vi "Startup.vi"(6 "Config":refnum<class "Config.lvclass">, 7 "Application":refnum<class "Application.lvclass">, 8 "error in (no error)":errorcluster, 9 "Log_Engine":refnum<class "Log_Engine.lvclass">, 10 "DAQ_Engine":refnum<class "DAQ_Engine.lvclass">, 11 "Main in":refnum<class "Main.lvclass">) -> (0 "error out":errorcluster, 3 "Main out":refnum<class "Main.lvclass">, 5 "Application out":refnum<class "Application.lvclass">)   [LabVIEW 2019, in "Main.lvclass"]
doc: "Developed by Kevin Thompson\nkevin@thompsonengineering.net\n\nCopyright 2018\nThompson Engineering, LLC"
uses:
  Main.lvclass
  Config/Config.lvclass
  Application/Application.lvclass
  DAQ_Engine/DAQ_Engine.lvclass
  Log_Engine/Log_Engine.lvclass
  DataTypes/Dependency--cluster.ctl
  Application/Application.lvclass/Application.ctl
  Config/Config.lvclass/Config.ctl
  Main.lvclass/Main.ctl
  Application/Accessors/Get InvWfmsQRef.vi
  Application/Accessors/Get PublicEvents.vi
  Application/Accessors/Get RawDaqDataQRef.vi
  Config/Accessors/Get Main Settings.vi
  Accessors/Set Dependency.vi
  Accessors/Set Settings.vi
  Accessors/Set InvWfmsQRef.vi
  Accessors/Set TerminateAppEvent.vi
  Accessors/Set RawDaqDataQRef.vi
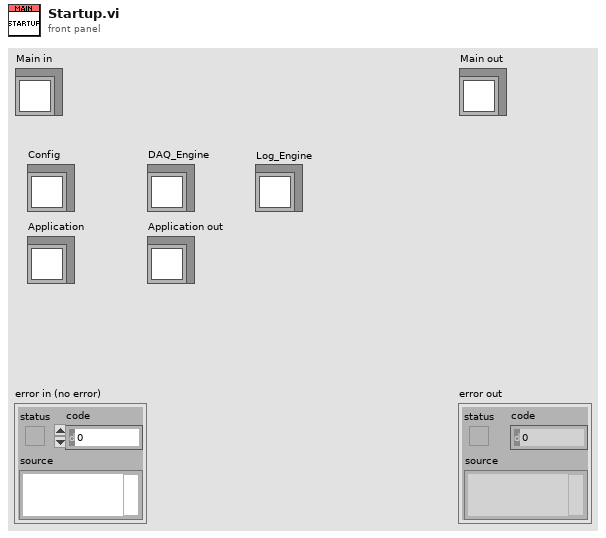
[diagram p1: front panel]
types:
  T1 = typedef "Main.lvclass/Dependency--cluster.ctl" = cluster{"Config":refnum<class "Config.lvclass">, "DAQ":refnum<class "DAQ_Engine.lvclass">, "Log_Engine":refnum<class "Log_Engine.lvclass">}
  T2 = typedef "InverterWaveforms--QRef.ctl" = refnum<queue>
  T3 = typedef "Application.lvclass/Public Events--cluster.ctl" = cluster{"Application.AsyncCmd Event":refnum<user-event>, "Application.AsyncMsg Event":refnum<user-event>, "stop process":refnum<user-event>}
  T4 = typedef "RawDAQDataQRef--cluster.ctl" = refnum<queue>
  T5 = typedef "Main.lvclass/Settings--cluster.ctl" = cluster{"Simulation":bool, "Signal scaling":T6[], "ESR scaling":T7[], "num readings to average":i32[], "ESR alarm threshhold (%)":i32[], "UseDummyVrms":bool, "Dummy Vrms":dbl, "Inverter Database File":path, "default Inverter (name)":string[]}
  T6 = typedef "Main.lvclass/Gain control.ctl" = cluster{"Iin ripple gain":dbl, "Iout ripple gain":dbl, "Iout 60Hz gain ":dbl, "Vout 60Hz gain ":dbl, "Iin ripple offest":dbl, "Iout ripple offset":dbl, "Iout 60Hz offset":dbl, "Vout 60Hz offset":dbl}
  T7 = typedef "Main.lvclass/ESR scaling--cluster.ctl" = cluster{"Gain":dbl, "Offset":dbl}
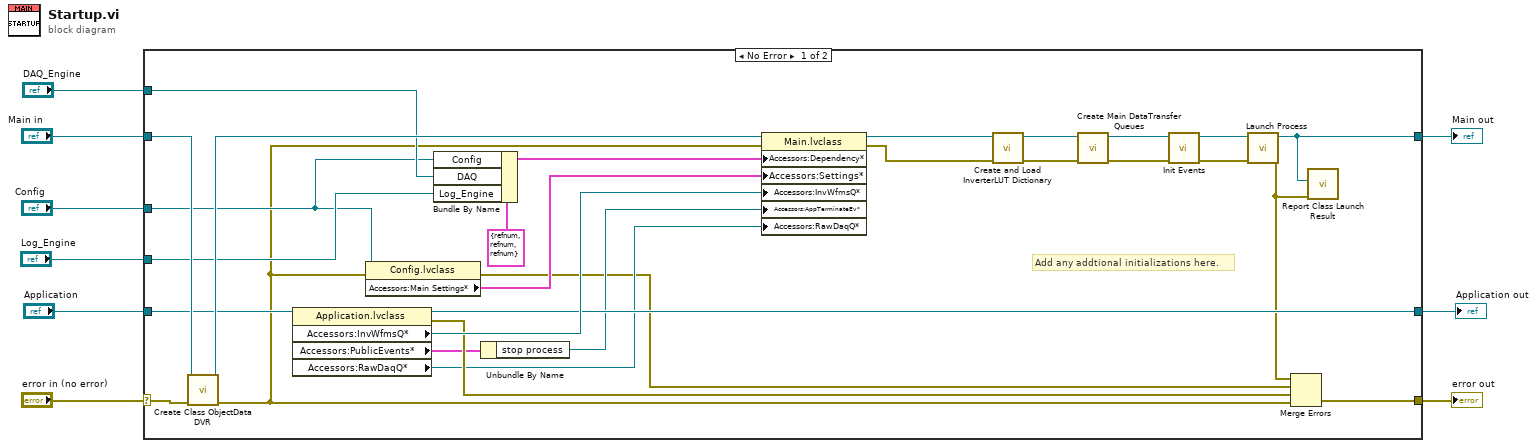
[diagram p0: block diagram]
diagram:
  n1 = case shown="No Error" "error in (no error)" {
    selector: "error in (no error)" -> [w38 w41]
    tunnel: [w35 w41] -> w8
    tunnel: [w24 w40] -> w6
    tunnel: "Main in" -> [w37 w40]
    tunnel: "Config" -> [w19 _]
    tunnel: "Application" -> [w33 w39]
    tunnel: [w30 w39] -> w3
    tunnel: "DAQ_Engine" -> [w28 _]
    tunnel: "Log_Engine" -> [w27 _]
    frame No Error {
      # "Add any addtional initializations here."
      n2 = call "Create Class ObjectData DVR.vi"("error in (no error)"=w38, "Main in"=w37) -> ("error out"=w17:errorcluster, "Main out"=w36:refnum<class "Main.lvclass">)  [unwired: 8 in]
      n3 = property class="Application.lvclass"(reference=w33) -> (reference out=w30:refnum<class "Application.lvclass">, error out=w31:errorcluster, "Accessors:InvWfmsQ*"=w32:T2, "Accessors:PublicEvents*"=w26:T3, "Accessors:RawDaqQ*"=w22:T4)  [unwired: 1 in]
      n4 = property class="Config.lvclass"(reference=w19, error in=w17) -> (error out=w16:errorcluster, "Accessors:Main Settings*"=w18:T5)  [unwired: 1 out]
      n5 = Bundle By Name(cluster=T1 {"Config"=refnum, "DAQ"=refnum, "Log_Engine"=refnum} ("Dependency"), "Config"=w19, "DAQ"=w28, "Log_Engine"=w27) -> (w29:T1)
      n6 = Unbundle By Name(w26) -> ("stop process"=w25:refnum<user-event>)
      n7 = property class="Main.lvclass"(reference=w36, error in=w17, "Accessors:Dependency*"=w29, "Accessors:Settings*"=w18, "Accessors:InvWfmsQ*"=w32, "Accessors:AppTerminateEv*"=w25, "Accessors:RawDaqQ*"=w22) -> (reference out=w13:refnum<class "Main.lvclass">, error out=w11:errorcluster)
      n8 = call "Create and Load InverterLUT Dictionary.vi"("error in (no error)"=w11, "Main.lvclass"=w13) -> ("error out"=w10:errorcluster, "Main out"=w12:refnum<class "Main.lvclass">)  [unwired: 8 in]
      n9 = call "Create Main DataTransfer Queues.vi"("error in (no error)"=w10, "Main in"=w12) -> ("error out"=w20:errorcluster, "Main out"=w21:refnum<class "Main.lvclass">)  [unwired: 6 in, 2 out]
      n10 = call "Init Events.vi"("error in (no error)"=w20, "Main in"=w21) -> ("error out"=w15:errorcluster, "Main out"=w14:refnum<class "Main.lvclass">)  [unwired: 8 in]
      n11 = call "Launch Process.vi"("error in (no error)"=w15, "Main in"=w14) -> ("error out"=w23:errorcluster, "Main out"=w24:refnum<class "Main.lvclass">)  [unwired: 6 in, 2 out]
      n12 = Merge Errors(w23, w16, w31, w17) -> (w35:errorcluster)
      n13 = call "Report Class Launch Result.vi"("Object"=w24, "error in (no error)"=w23) -> ()  [unwired: 8 in, 1 out]
    }
    frame Error {
    }
  }
  "error out" <- w8
  "Main out" <- w6
  "Application out" <- w3
